vi "Memory.Move.vi"(8 "error in (no error)":errorcluster, 9 "size":i64 format="%d bytes", 10 "dst address":u64 format="%016x", 11 "src address":u64 format="%016x") -> (0 "error out":errorcluster)   [LabVIEW 2016, in "LabVIEW Memory Manager.lvlib"]
uses:
  LabVIEW Memory Manager.lvlib
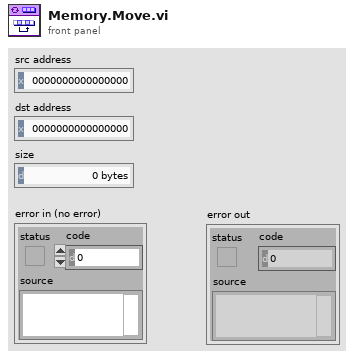
[diagram p1: front panel]
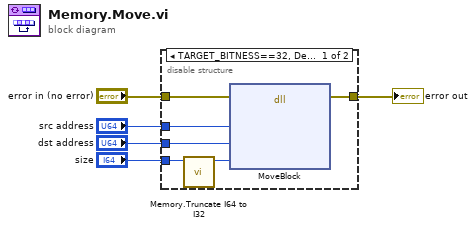
[diagram p0: block diagram]
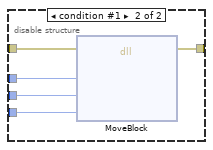
[diagram p2: hidden frame]
diagram:
  n1 = disable-structure shown="TARGET_BITNESS==32, Default" {
    disable-tunnel: "size" -> [w11 w13]
    disable-tunnel: "error in (no error)" -> [w10 w16]
    disable-tunnel: [w8 w14] -> w3
    disable-tunnel: "src address" -> [w9 w15]
    disable-tunnel: "dst address" -> [w6 w12]
    frame condition #0 (active) {
      n2 = call "Memory.Truncate I64 to I32.vi"("I64"=w11) -> ("truncated I32"=w7:i32)  [unwired: 10 in]
      n3 = dll-call lib="LabVIEW" fn="MoveBlock"(error in=w10, "src"=w9, "dst"=w6, "size"=w7) -> (error out=w8:errorcluster)  [unwired: 6 in, 1 out]
    }
    frame condition #1 {
      n4 = dll-call lib="LabVIEW" fn="MoveBlock"(error in=w16, "src"=w15, "dst"=w12, "size"=w13) -> (error out=w14:errorcluster)  [unwired: 6 in, 1 out]
    }
  }
  "error out" <- w3
